vi "复位结果.vi"   [LabVIEW 2014]
uses:
  <vilib>/Modbus/master/Create Master Instance (Serial).vi
  <vilib>/Modbus/master/Modbus Master.lvclass
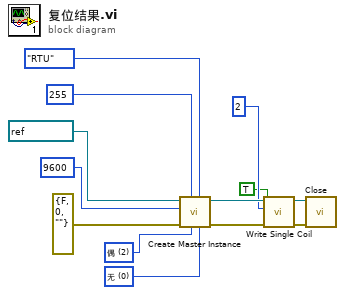
[diagram p0: block diagram]
diagram:
  w11 = u16 2 items=["无", "奇", "偶"] ("parity (Even)")
  w13 = u16 0 items=["无", "XON/XOFF", "RTS/CTS", "XON/XOFF & RTS/CTS", "DTR/DSR", "XON/XOFF & DTR/DSR"] ("flow control (None)")
  n1 = call-poly <vilib>:"Create Master Instance.vi"("flow control (None)"=w13, "serial type"=enum16{"RTU", "ASCII"}."RTU", "parity (Even)"=w11, "unit ID"=u8 255, "error in (no error)"=errorcluster {"status"=FALSE, "code"=0, "source"=""}, "baud rate (9600)"=u32 9600, "VISA resource name"=refnum<visa-resource-name> "COM7") -> ("error out"=w5:errorcluster, "serial master instance"=w6:refnum<class "Modbus Master.lvclass">)  [unwired: 3 in]
  n2 = call-dynamic "Write Single Coil.vi"("error in (no error)"=w5, "coil value"=TRUE, "address"=u16 2, "Modbus master in"=w6) -> ("error out"=w2:errorcluster, "Modbus master out"=w3:refnum<class "Modbus Master.lvclass">)  [unwired: 6 in]
  n3 = call-dynamic "Close.vi"("error in (no error)"=w2, "Modbus master in"=w3) -> ()  [unwired: 9 in, 1 out]
